vi "Build Tree.vi"(5 "Defer Updates (T)":bool=TRUE, 7 "Tree":refnum<vi>, 8 "error in":errorcluster, 10 "Blacklist":set{string}(c389), 11 "Tree Map in":refnum<class "Tree Map.lvclass">) -> (0 "error out":errorcluster, 3 "Tree Map out":refnum<class "Tree Map.lvclass">)   [LabVIEW 2020, in "VI Properties Editor.lvlib" / "Tree Map.lvlib" / "Tree Map.lvclass"]
uses:
  Tree Map.lvclass
  Tree Map.lvclass/Tree Map.ctl
  Tree Map.lvlib
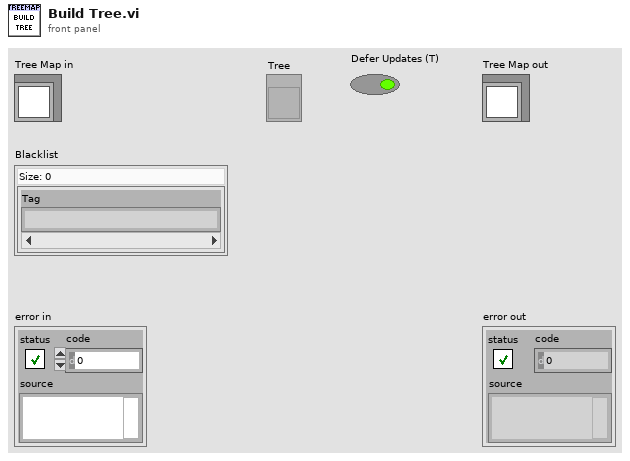
[diagram p1: front panel]
types:
  T1 = typedef "LVNodeAndColumnTypeDef.ctl" = cluster{"Node":string, "Column":i32}
  T2 = typedef "VI Properties Editor.lvlib/Tree Map.lvlib/Tree Map.lvclass/Tree Entry.ctl" = cluster{"Hierarchy":string[], "Name":string, "Columns":string[], "BG Color":u32, "Leaf":bool, "Symbol":string}
  T3 = typedef "imagedata.ctl" = cluster{"image type":i32, "image depth":i32, "image":u8[], "mask":u8[], "colors":u32[], "Rectangle":cluster{"left":i16, "top":i16, "right":i16, "bottom":i16}}
  T4 = map{string, cluster{"index":i32, "image data":T3}}
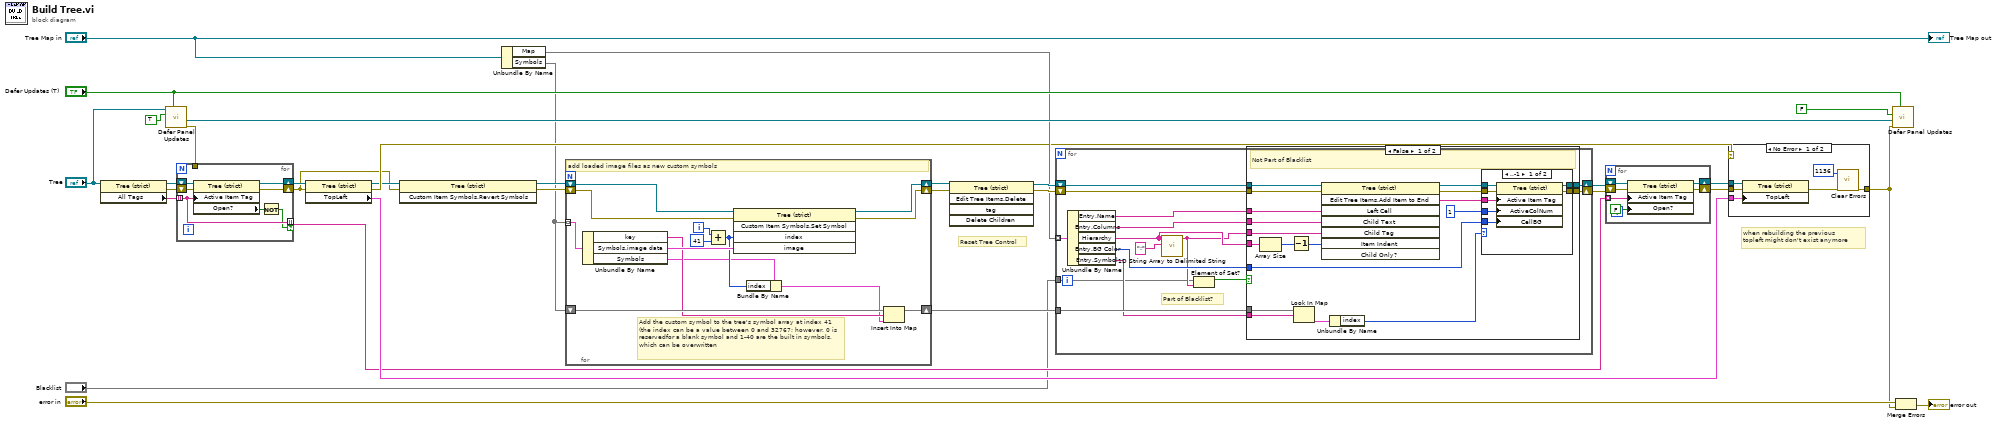
[diagram p0: block diagram]
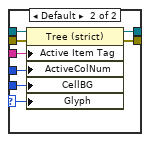
[diagram p2: hidden frame]
diagram:
  # "when rebuilding the previous\ntopleft might don't exist anymore"
  # "Reset Tree Control"
  n1 = property class="Tree (strict)"(reference="Tree") -> (reference out=w28:refnum<vi>, error out=w15:errorcluster, "All Tags"=w29:string[])  [unwired: 1 in]
  n2 = call "Defer Panel Updates.vi"("Set Defer (T)"="Defer Updates (T)", "Defer"=TRUE, "Tree (Front Panel)"="Tree") -> ("error out"=w16:errorcluster, "Front Panel"=w20:refnum<vi>)  [unwired: 7 in]
  n3 = for {
    tunnel: w29 -> [w38] mode=indexing
    shift-right: [w36] -> w27
    shift-left: w28 -> [w40]
    tunnel: [w38] -> w26 mode=indexing if=w37
    tunnel: w16 -> [_]
    shift-right: [w34] -> w6
    shift-left: w15 -> [w35]
    n4 = property class="Tree (strict)"(reference=w40, error in=w35, "Active Item Tag"=w38) -> (reference out=w36:refnum<vi>, error out=w34:errorcluster, "Open?"=w39:bool)
    n5 = Not(x=w39) -> (.not. x?=w37:bool)
  }
  n6 = property class="Tree (strict)"(reference=w27, error in=w6) -> (reference out=w9:refnum<vi>, error out=w10:errorcluster, "TopLeft"=w30:T1)
  n7 = invoke on="Invoke Node" class="Tree (strict)" method="Custom Item Symbols.Revert Symbols"(reference=w9, error in=w6) -> (reference out=w8:refnum<vi>, error out=w7:errorcluster)  [unwired: 1 in, 1 out]
  n8 = Unbundle By Name("Tree Map in") -> ("Map"=w17:map{string[], T2}, "Symbols"=w4:T4)
  n9 = for {
    shift-right: [w52] -> w2
    shift-left: w8 -> [w54]
    shift-right: [w51] -> w5
    shift-left: w7 -> [w53]
    tunnel: w4 -> [w47] mode=indexing
    shift-right: [w43] -> w3
    shift-left: w4 -> [w45]
    i -> [w50]
    # "Add the custom symbol to the tree's symbol array at index 41 (the index can be a value between 0 and 32767; however, 0 is reservedfor a blank symbol and 1-40 are the built in symbols, which can be overwritten"
    # "add loaded image files as new custom symbols"
    n10 = Unbundle By Name(w47) -> ("key"=w44:string, "Symbols.image data"=w49:T3, "Symbols"=w41:cluster{"index":i32, "image data":T3})
    n11 = Add(x=w50, y=41 ("Index")) -> (x+y=w46:i32)
    n12 = invoke on="Invoke Node" class="Tree (strict)" method="Custom Item Symbols.Set Symbol"(reference=w54, error in=w53, "index"=w46, "image"=w49) -> (reference out=w52:refnum<vi>, error out=w51:errorcluster)  [unwired: 1 in, 3 out]
    n13 = Bundle By Name(cluster=w41, "index"=w46) -> (w42:cluster{"index":i32, "image data":T3})
    n14 = Insert Into Map(map in=w45, key=w44, value=w42) -> (map out=w43:T4)  [unwired: 2 out]
  }
  n15 = invoke class="Tree (strict)" method="Edit Tree Items.Delete"(reference=w2, error in=w5) -> (reference out=w31:refnum<vi>, error out=w33:errorcluster)  [unwired: 3 in, 3 out]
  n16 = for {
    shift-right: [w62] -> w24
    shift-left: w31 -> [w69]
    tunnel: w17 -> [w63] mode=indexing
    shift-right: [w61] -> w14
    shift-left: w33 -> [w65]
    tunnel: w3 -> [w60]
    tunnel: "Blacklist" -> [w56]
    # "Part of Blacklist?"
    n17 = Unbundle By Name(w63) -> ("Entry.Name"=w66:string, "Entry.Columns"=w67:string[], "Hierarchy"=w64:string[], "Entry.BG Color"=w58:u32, "Entry.Symbol"=w59:string)
    n18 = call <vilib>:"1D String Array to Delimited String.vi"("delimiter"=":", "string array"=w64) -> ("delimited string"=w57:string)  [unwired: 9 in]
    n19 = Element of Set?(10:w57, 11:w56) -> (3:w55:bool)
    n20 = case shown="False" w55 {
      tunnel: w69 -> [w88 w104]
      tunnel: w57 -> [w87 _]
      tunnel: w67 -> [w84 _]
      tunnel: w66 -> [w83 _]
      tunnel: w65 -> [w82 w105]
      tunnel: w64 -> [w81 _]
      tunnel: [w76 w104] -> w62
      tunnel: [w75 w105] -> w61
      tunnel: w60 -> [w74 _]
      tunnel: w59 -> [w71 _]
      tunnel: w58 -> [w70 _]
      frame False {
        # "Not Part of Blacklist"
        n21 = Array Size(array=w81) -> (size(s)=w86:i32)
        n22 = Decrement(x=w86) -> (x-1=w85:i32)
        n23 = Look In Map(map=w74, key=w71) -> (value=w73:cluster{"index":i32, "image data":T3})  [unwired: 1 in, 1 out]
        n24 = invoke class="Tree (strict)" method="Edit Tree Items.Add Item to End"(reference=w88, error in=w82, "Left Cell"=w83, "Child Text"=w84, "Child Tag"=w87, "Item Indent"=w85) -> (reference out=w80:refnum<vi>, error out=w79:errorcluster, "Edit Tree Items:Add Item to End"=w78:string)  [unwired: 2 in, 5 out]
        n25 = Unbundle By Name(w73) -> ("index"=w72:i32)
        n26 = case shown="..-1" w72 {
          selector: w72 -> [_ w96]
          tunnel: w80 -> [w94 w103]
          tunnel: w79 -> [w95 w102]
          tunnel: w78 -> [w89 w101]
          tunnel: 1 ("Active Cell:Active Column Number") -> [w90 w100]
          tunnel: [w92 w99] -> w76
          tunnel: [w93 w98] -> w75
          tunnel: w70 -> [w91 w97]
          frame ..-1 {
            n27 = property class="Tree (strict)"(reference=w94, error in=w95, "Active Item Tag"=w89, "ActiveColNum"=w90, "CellBG"=w91) -> (reference out=w92:refnum<vi>, error out=w93:errorcluster)
          }
          frame Default {
            n28 = property class="Tree (strict)"(reference=w103, error in=w102, "Active Item Tag"=w101, "ActiveColNum"=w100, "CellBG"=w97, "Glyph"=w96) -> (reference out=w99:refnum<vi>, error out=w98:errorcluster)
          }
        }
      }
      frame True {
        # "Part of Blacklist"
      }
    }
  }
  n29 = for {
    shift-right: [w110] -> w25
    shift-left: w24 -> [w111]
    tunnel: w26 -> [w108] mode=indexing
    shift-right: [w106] -> w13
    shift-left: w14 -> [w107]
    n30 = property class="Tree (strict)"(reference=w111, error in=w107, "Active Item Tag"=w108, "Open?"=FALSE ("Active Item:Open?")) -> (reference out=w110:refnum<vi>, error out=w106:errorcluster)
  }
  n31 = case shown="No Error" w10 {
    tunnel: w30 -> [w117 _]
    tunnel: w25 -> [w116 _]
    tunnel: w13 -> [w115 w118]
    tunnel: [w113 w118] -> w11
    frame No Error {
      n32 = property class="Tree (strict)"(reference=w116, error in=w115, "TopLeft"=w117) -> (error out=w114:errorcluster)  [unwired: 1 out]
      n33 = call <vilib>:"Clear Errors.vi"("error in (no error)"=w114, "specific error code to clear (0: all)"=1136) -> ("error out"=w113:errorcluster)  [unwired: 4 in, 1 out]
    }
    frame Error {
    }
  }
  n34 = call "Defer Panel Updates.vi"("Set Defer (T)"="Defer Updates (T)", "error in (no error)"=w11, "Front Panel (Lookup)"=w20, "Defer"=FALSE ("Defer Panel Updates")) -> ()  [unwired: 6 in, 2 out]
  n35 = Merge Errors("error in", w11) -> (→"error out":errorcluster)
  "Tree Map out" <- "Tree Map in"
